vi "Summarise.vi"(0 "Channel Names":string[](array[string]), 1 "Data":string[][](array[string]), 3 "Summarise All":bool) -> (5 "Summary":string[][](array[string]))   [LabVIEW 2020]
uses:
  Results_plotter_Global.vi
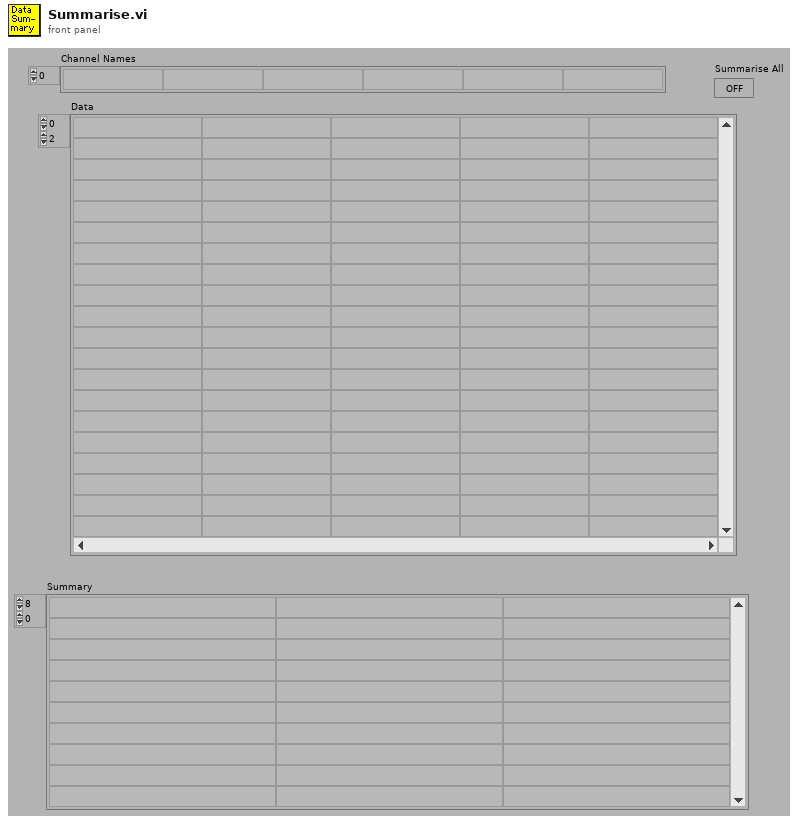
[diagram p1: front panel]
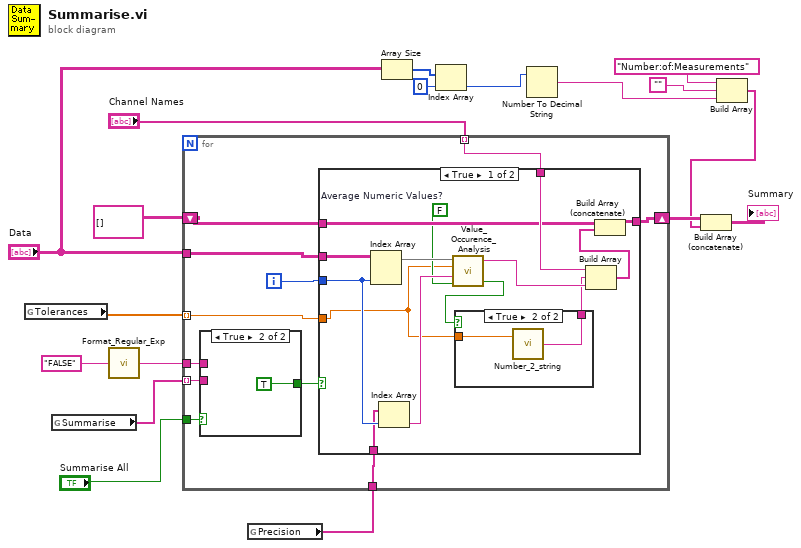
[diagram p0: block diagram]
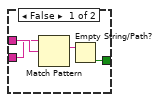
[diagram p2: hidden frame]
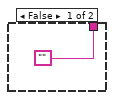
[diagram p3: hidden frame]
diagram:
  n1 = global read "Results_plotter_Global.vi" "Tolerances"() -> (w15:dbl[])
  n2 = global read "Results_plotter_Global.vi" "Summarise"() -> (w12:string[])
  n3 = call "Format_Regular_Exp.vi"("Regular expression"="FALSE" ("y")) -> ("Case Insensitive for html"=w13:string)
  n4 = global read "Results_plotter_Global.vi" "Precision"() -> (w16:string[])
  n5 = for {
    tunnel: "Data" -> [w29]
    tunnel: w15 -> [w26] mode=indexing
    tunnel: "Channel Names" -> [w27] mode=indexing
    shift-right: [w24] -> w2
    shift-left: string[][] [] -> [w25]
    tunnel: w16 -> [w23]
    tunnel: w13 -> [w22]
    tunnel: w12 -> [w21] mode=indexing
    tunnel: "Summarise All" -> [w20]
    i -> [w28]
    n6 = case shown="True" w20 {
      tunnel: w22 -> [w33 _]
      tunnel: w21 -> [w32 _]
      tunnel: [w30 TRUE] -> w19
      frame False {
        n7 = Match Pattern(string=w32, regular expression=w33) -> (match substring=w31:string)  [unwired: 4 out]
        n8 = Empty String/Path?(string/path=w31) -> (empty?=w30:bool)
      }
      frame True {
      }
    }
    n9 = case shown="True" w19 {
      tunnel: w29 -> [w48 _]
      tunnel: w28 -> [w39 _]
      tunnel: w27 -> [w46 _]
      tunnel: w26 -> [w35 _]
      tunnel: w25 -> [w44 w52]
      tunnel: [w43 w52] -> w24
      tunnel: w23 -> [w38 _]
      frame True {
        w36 = FALSE  # Average Numeric Values?
        n10 = Index Array(array=w48, index (col)=w39) -> (element=w47:string[])  [unwired: 1 in]
        n11 = Index Array(array=w38, index=w39) -> (element=w37:string)
        n12 = call "Value_Occurence_Analysis.vi"("Average Numeric Values?"=w36, "Tolerance"=w35, "Precision (3)"=w37, "String Array"=w47) -> ("Numeric Array?"=w40:bool, "Output String"=w45:string)  [unwired: 1 out]
        n13 = case shown="True" w40 {
          tunnel: w35 -> [_ w51]
          tunnel: ["" w50] -> w41
          frame False {
          }
          frame True {
            n14 = call "Number_2_string.vi"("number"=w51) -> ("String"=w50:string)  [unwired: 1 in]
          }
        }
        n15 = Build Array(w46, w41, w45) -> (w42:string[])
        n16 = Build Array (concatenate)(w44, w42) -> (w43:string[][])
      }
      frame False {
      }
    }
  }
  n17 = Array Size(array="Data") -> (size(s)=w9:i32[])
  n18 = Index Array(array=w9, index=0) -> (element=w7:i32)
  n19 = Number To Decimal String(number=w7) -> (decimal integer string=w5:string)  [unwired: 1 out]
  n20 = Build Array("Number:of:Measurements", "", w5) -> (w1:string[])
  n21 = Build Array (concatenate)(w2, w1) -> (→"Summary":string[][])
